vi "intCSMs.vi"(8 "error in (no error)":errorcluster, 11 "TestCase in":refnum<class "testcase-CSMSubModule.lvclass">) -> (0 "error out":errorcluster, 3 "TestCase out":refnum<class "testcase-CSMSubModule.lvclass">)   [LabVIEW 2017, in "testcase-CSMSubModule.lvclass"]
uses:
  testcase-CSMSubModule.lvclass
  src/user.lib/_NEVSTOP/Communicable State Machine(CSM)/_Support/Typedef/_CSM_List Module Scope.ctl
  testcase-CSMSubModule.lvclass/testcase-CSMSubModule.ctl
  CSM/Normal-CSM.vi
  CSM/CSM-Testcase.lvlib
  src/user.lib/_NEVSTOP/Communicable State Machine(CSM)/Communicable State Machine.lvlib
panel:
  out "Module Names":string[](array[string])
  out "CSMs Left":string[](array[string])
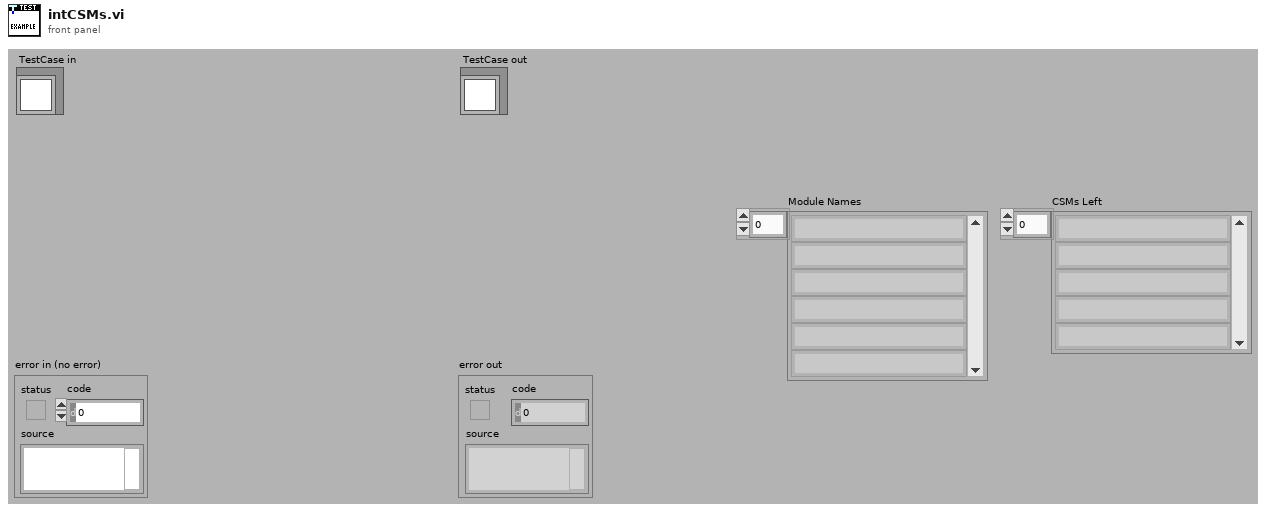
[diagram p1: front panel]
types:
  T1 = typedef "Communicable State Machine.lvlib/_CSM_List Module Scope.ctl" = enum16{"Normal", "System Only", "All"}
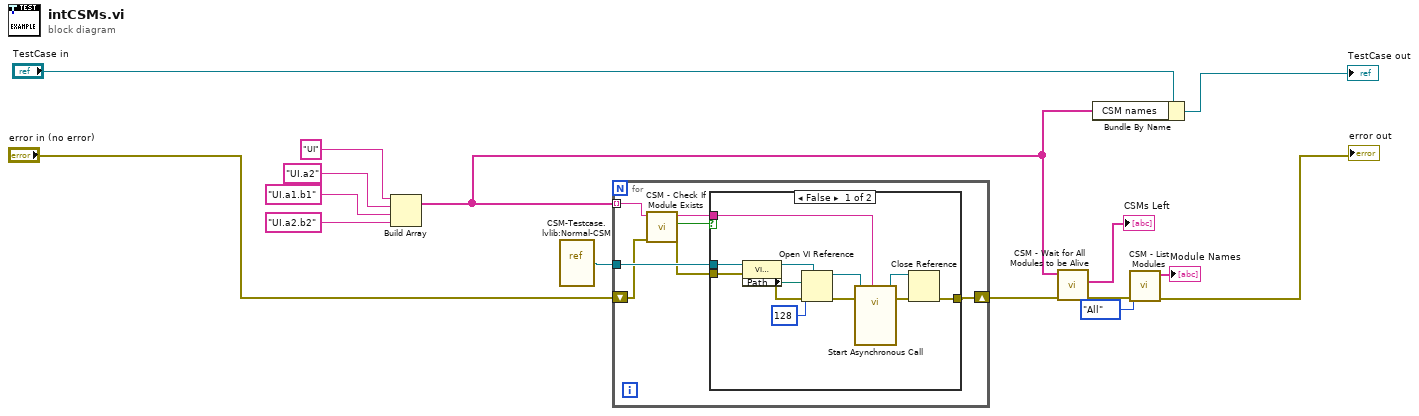
[diagram p0: block diagram]
diagram:
  n1 = Build Array("UI" ("Name (\"\" to Use UUID)"), "UI.a2" ("Name (\"\" to Use UUID)"), "UI.a1.b1" ("Name (\"\" to Use UUID)"), "UI.a2.b2" ("Name (\"\" to Use UUID)")) -> (w1:string[])
  n2 = vi-ref "CSM-Testcase.lvlib:Normal-CSM.vi"() -> (w13:refnum<vi>)
  n3 = for {
    tunnel: w13 -> [w22]
    tunnel: w1 -> [w19] mode=indexing
    shift-right: [w16] -> w10
    shift-left: "error in (no error)" -> [w21]
    n4 = call "CSM - Check If Module Exists.vi"("Error In"=w21, "CSM Name"=w19) -> ("error out"=w20:errorcluster, "Exist?"=w17:bool, "CSM Name (Dup)"=w18:string)  [unwired: 7 in]
    n5 = case shown="False" w17 {
      tunnel: w22 -> [w26 _]
      tunnel: [w25 w35] -> w16
      tunnel: w20 -> [w24 w35]
      tunnel: w18 -> [w23 _]
      frame False {
        n6 = property class="VI (strict)"(reference=w26, error in=w24) -> (reference out=w32:refnum<vi>, error out=w30:errorcluster, "Path"=w29:path)
        n7 = Open VI Reference(type specifier VI Refnum (for type only)=w32, vi path=w29, options=128, error in (no error)=w30) -> (vi reference=w28:refnum<vi>, error out=w33:errorcluster)  [unwired: 2 in]
        n8 = call-by-ref "Start Asynchronous Call"(reference=w28, error in=w33, "Name (\"\" to Use UUID)"=w23) -> (reference out=w27:refnum<vi>, error out=w31:errorcluster)  [unwired: 11 in]
        n9 = Close Reference(reference=w27, error in (no error)=w31) -> (error out=w25:errorcluster)
      }
      frame True {
      }
    }
  }
  n10 = call "CSM - Wait for All Modules to be Alive.vi"("Error In"=w10, "CSM Names"=w1) -> ("error out"=w8:errorcluster, "CSMs Left"=→"CSMs Left":string[])  [unwired: 7 in, 1 out]
  n11 = Bundle By Name(cluster="TestCase in", "CSM names"=w1) -> (→"TestCase out":refnum<class "testcase-CSMSubModule.lvclass">)
  n12 = call "CSM - List Modules.vi"("Error In"=w8, "Scope (Normal)"=_CSM_List_Module_Scope."All") -> ("error out"=→"error out":errorcluster, "Module Names"=→"Module Names":string[])  [unwired: 8 in]
